vi "WPI_CameraGetScaledAttr.vi"(7 "Attr Format":string="CameraAttributes::%s::Value", 8 "error in (no error)":errorcluster, 10 "Attr String":string, 11 "Camera Address In":string) -> (0 "error out":errorcluster, 1 "Raw":dbl, 2 "Scaled":dbl, 3 "Camera Address Out":string)   [LabVIEW 2017]
doc: "Returns the scaled and raw value of a numeric camera attribute.\n\n\nThis software is licensed. Open the labview\\readme\\WPI Robotics Library Open Source License.txt file for more information."
uses:
  <vilib>/userdefined/High Color/IMAQdx.ctl
  <resource>/objmgr/imaqdx.rc
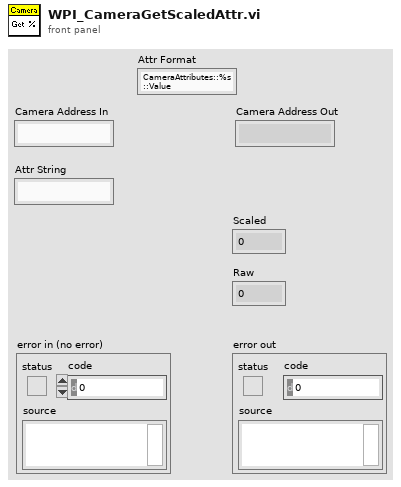
[diagram p1: front panel]
types:
  T1 = typedef "IMAQdx.ctl" = refnum<k21>
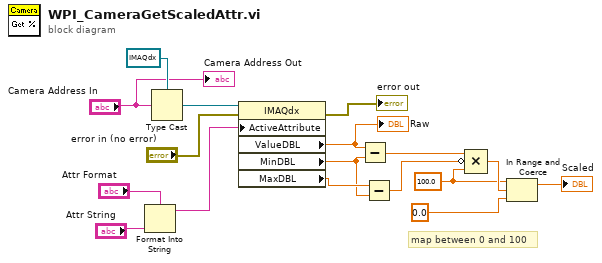
[diagram p0: block diagram]
diagram:
  w5 = 100.0
  # "map between 0 and 100"
  n1 = Format Into String(format string="Attr Format", "Attr String") -> (resulting string=w13:string)  [unwired: 2 in, 1 out]
  n2 = Type Cast(type=T1 refnum ("Session In"), x="Camera Address In") -> (*(type *) &x=w16:T1)
  n3 = property class="IMAQdx"(reference=w16, error in="error in (no error)", "ActiveAttribute"=w13) -> (error out=→"error out":errorcluster, "ValueDBL"=w11:dbl, "MinDBL"=w9:dbl, "MaxDBL"=w10:dbl)  [unwired: 1 out]
  "Raw" <- w11
  n4 = Subtract(x=w11, y=w9) -> (x-y=w8:dbl)
  n5 = Subtract(x=w10, y=w9) -> (x-y=w7:dbl)
  n6 = Compound Arithmetic op=MULTIPLY(w8, invert w7, w5) -> (w6:dbl)
  n7 = In Range and Coerce(upper limit=w5, x=w6, lower limit=0.0) -> (coerced(x)=→"Scaled":dbl)  [unwired: 1 out]
  "Camera Address Out" <- "Camera Address In"
